vi "Pneumatic gripper Relax.vi"(8 "error in":errorcluster) -> (0 "error out":errorcluster)   [LabVIEW 2019]
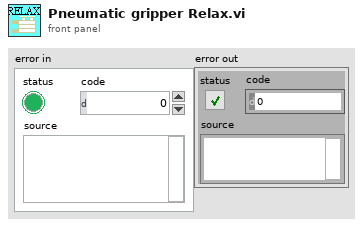
[diagram p1: front panel]
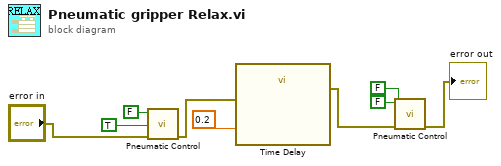
[diagram p0: block diagram]
diagram:
  n1 = call "Pneumatic Control.vi"("error in"="error in", "DIR"=TRUE, "ENA"=FALSE) -> ("error out"=w2:errorcluster)  [unwired: 8 in]
  n2 = call "Time Delay"("error in (no error)"=w2, "Delay Time (s)"=0.2) -> ("error out"=w1:errorcluster)  [unwired: 9 in]
  n3 = call "Pneumatic Control.vi"("error in"=w1, "DIR"=FALSE, "ENA"=FALSE) -> ("error out"=→"error out":errorcluster)  [unwired: 8 in]
